vi "SCD - Trigger Sequence Generation - Complete Recipe.vi"(8 "error in":errorcluster, 9 "FPS":dbl=10.0 min=1.0 max=30.0 format="%0.2p", 10 "Modulation Cycles\nAt Each Wavelength":dbl=1.0 min=1.0 max=30.0 step=1.0, 11 "LCVR Voltages":dbl[][](array[numeric])=[[0.5, 0.6, 0.7, 0.8, 0.9]]) -> (0 "error out":errorcluster, 1 "LCVR Relaxtion Time":dbl=200.0 format="%#_13g", 3 "SCD Waveforms (Graph)":waveform(dbl)[](graph)=[{"t0"=timestamp(0 s since 1904-01-01), "dt"=0.000125, "Y"=array[4803 elements]}, {"t0"=timestamp(0 s since 1904-01-01), "dt"=0.000125, "Y"=array[4803 elements]}, {"t0"=timestamp(0 s since 1904-01-01), "dt"=0.000125, "Y"=array[4803 elements]}, {"t0"=timestamp(0 s since 1904-01-01), "dt"=0.000125, "Y"=array[4803 elements]}, {"t0"=timestamp(0 s since 1904-01-01), "dt"=0.000125, "Y"=array[4803 elements]}, {"t0"=timestamp(0 s since 1904-01-01), "dt"=0.000125, "Y"=array[4803 elements]}, {"t0"=timestamp(0 s since 1904-01-01), "dt"=0.000125, "Y"=array[4803 elements]}, {"t0"=timestamp(0 s since 1904-01-01), "dt"=0.000125, "Y"=array[4803 elements]}])   [LabVIEW 2014]
doc: "This VI creates the complete recipe Analog Output waveform set for multiple wavelengths. Each wavelength change in the recipe requies a new 200ms 'relaxation' time for the LCVR's to reach the required retardance value. Finally, this VI pre-pends an Andor Neo Camera \"Arming\" trigger pulse. This is required in a sequence based acquisition."
uses:
  <vilib>/Waveform/WDTOps.llb/WDT Index Channel DBL.vi
  <vilib>/Waveform/WDTOps.llb/WDT Append Waveforms DBL.vi
panel:
  out "SCD Waveforms (cluster)":waveform(dbl)[](array[waveform])=[{"t0"=timestamp(0 s since 1904-01-01), "dt"=0.000125, "Y"=array[4803 elements]}, {"t0"=timestamp(0 s since 1904-01-01), "dt"=0.000125, "Y"=array[4803 elements]}, {"t0"=timestamp(0 s since 1904-01-01), "dt"=0.000125, "Y"=array[4803 elements]}, {"t0"=timestamp(0 s since 1904-01-01), "dt"=0.000125, "Y"=array[4803 elements]}, {"t0"=timestamp(0 s since 1904-01-01), "dt"=0.000125, "Y"=array[4803 elements]}, {"t0"=timestamp(0 s since 1904-01-01), "dt"=0.000125, "Y"=array[4803 elements]}, {"t0"=timestamp(0 s since 1904-01-01), "dt"=0.000125, "Y"=array[4803 elements]}, {"t0"=timestamp(0 s since 1904-01-01), "dt"=0.000125, "Y"=array[4803 elements]}]
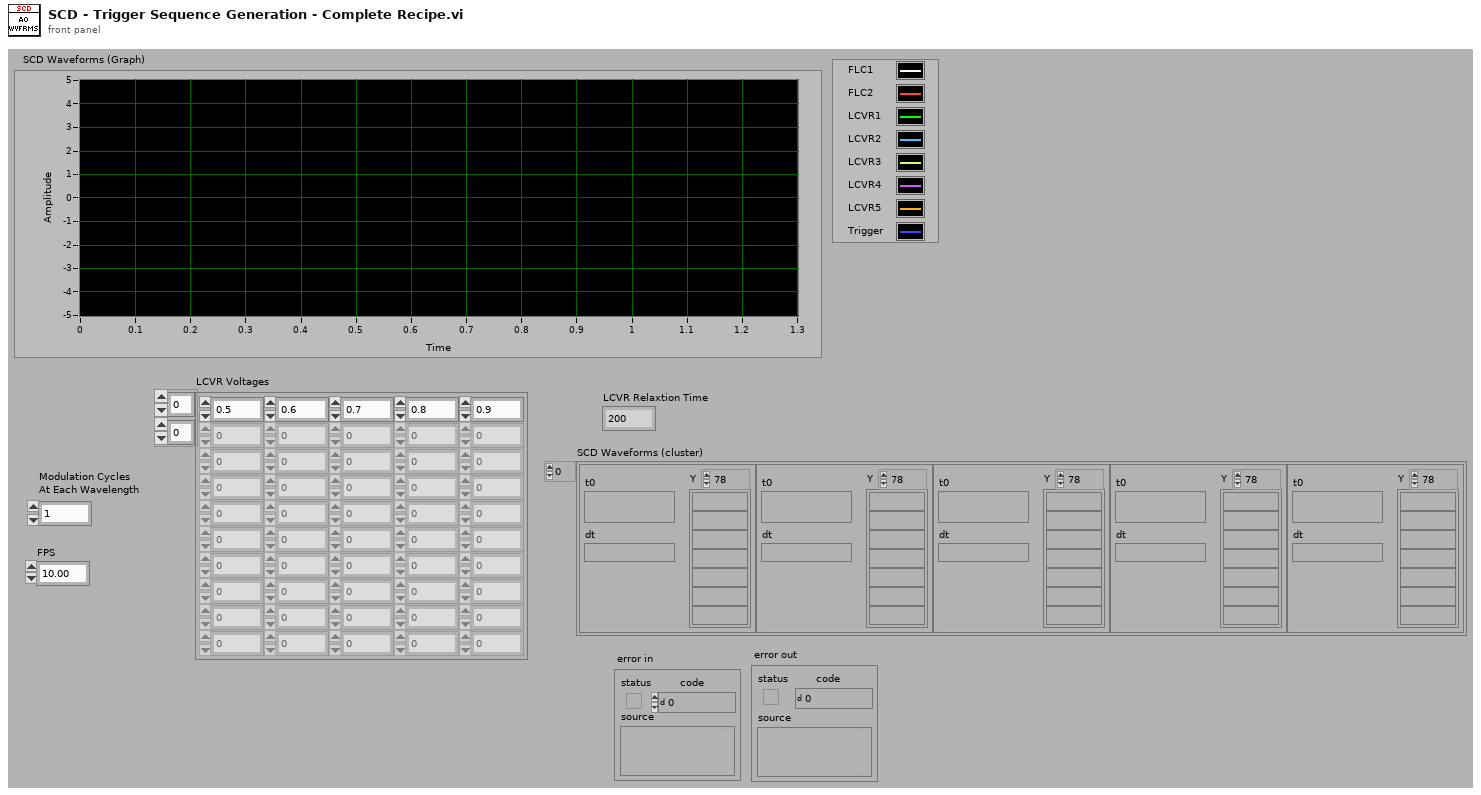
[diagram p1: front panel]
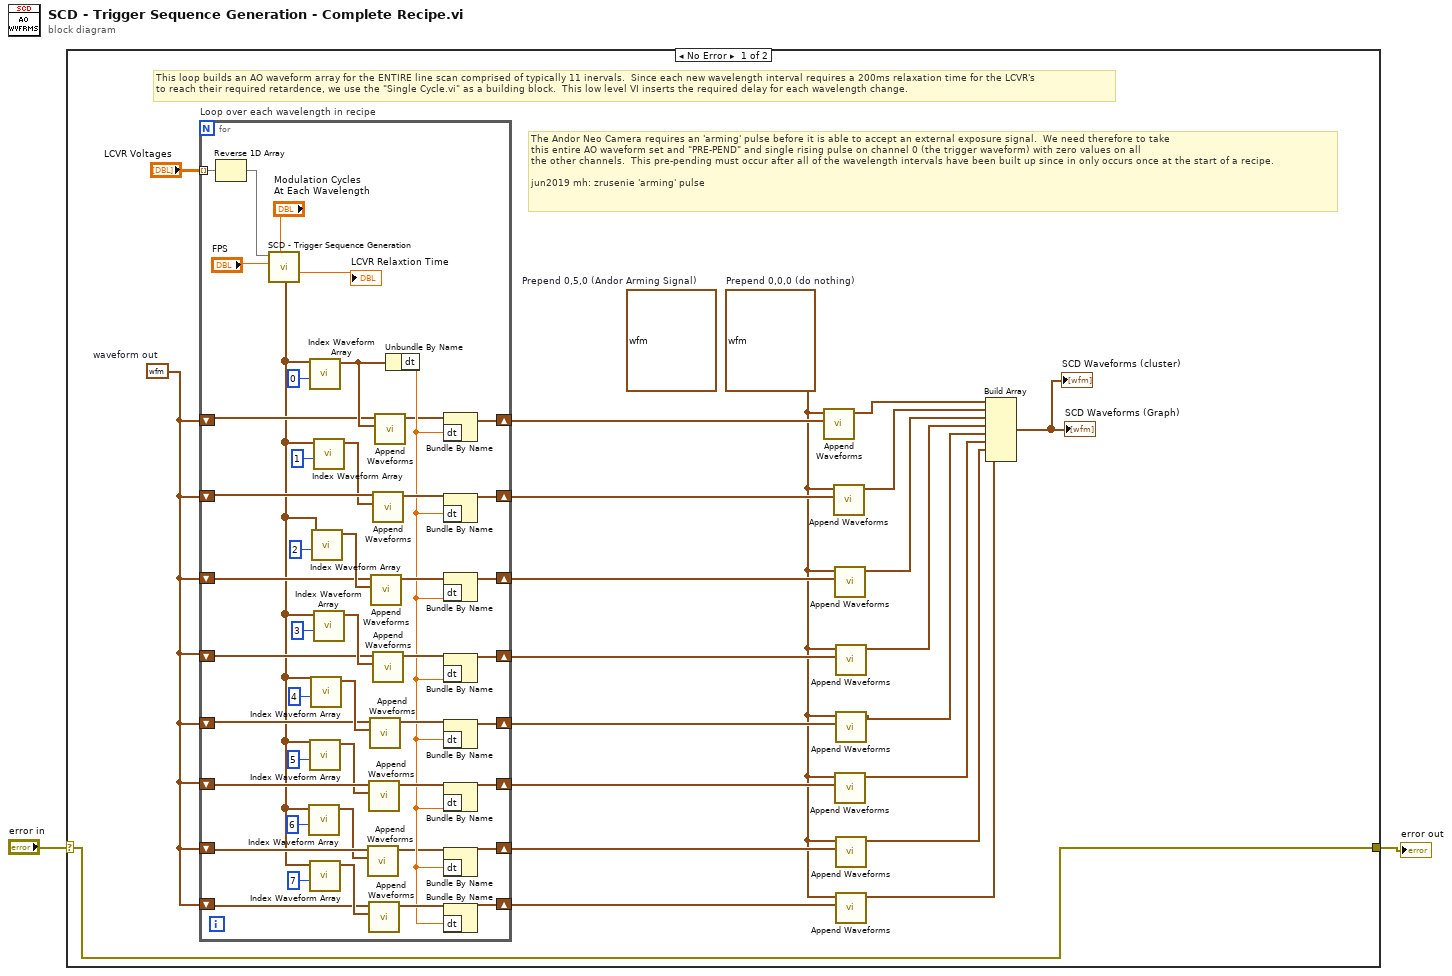
[diagram p0: block diagram]
diagram:
  n1 = case shown="No Error" "error in" {
    selector: "error in" -> [w6 w71]
    tunnel: [w6 w71] -> w1
    frame No Error {
      w3 = waveform(dbl) {"t0"=timestamp(0 s since 1904-01-01), "dt"=0.000125, "Y"=[0.0, 0.0, 0.0]}  # Prepend 0,0,0 (do nothing)
      (unwired) waveform(dbl) {"t0"=timestamp(0 s since 1904-01-01), "dt"=0.000125, "Y"=[0.0, 5.0, 0.0]}  # Prepend 0,5,0 (Andor Arming Signal)
      w23 = waveform(dbl) {"t0"=timestamp(0 s since 1904-01-01), "dt"=1.0, "Y"=[]}  # waveform out
      # "The Andor Neo Camera requires an 'arming' pulse before it is able to accept an external exposure signal.  We need therefore to take\nthis entire AO waveform set and \"PRE-PEND\" and single rising pulse on channel 0 (the trigger waveform) with zero values on all\nthe other channels.  This pre-pending must occur after all of the wavelength intervals have been built up since in only occurs once at the start of a recipe.\n\njun2019 mh: zrusenie 'arming' pulse"
      # "This loop builds an AO waveform array for the ENTIRE line scan comprised of typically 11 inervals.  Since each new wavelength interval requires a 200ms relaxation time for the LCVR's \nto reach their required retardence, we use the \"Single Cycle.vi\" as a building block.  This low level VI inserts the required delay for each wavelength change."
      n2 = for "Loop over each wavelength in recipe" {
        shift-right: [w43] -> w21
        shift-left: w23 -> [w33]
        shift-right: [w27] -> w20
        shift-left: w23 -> [w66]
        shift-right: [w44] -> w18
        shift-left: w23 -> [w53]
        shift-right: [w45] -> w10
        shift-left: w23 -> [w52]
        shift-right: [w46] -> w11
        shift-left: w23 -> [w51]
        shift-right: [w47] -> w15
        shift-left: w23 -> [w50]
        shift-right: [w48] -> w13
        shift-left: w23 -> [w32]
        shift-right: [w38] -> w12
        shift-left: w23 -> [w39]
        tunnel: "LCVR Voltages" -> [w26] mode=indexing
        n3 = Reverse 1D Array(array=w26) -> (reversed array=w36:dbl[])
        n4 = call "SCD - Trigger Sequence Generation.vi"("Modulation Cycles\n per Wavelength"="Modulation Cycles\nAt Each Wavelength", "FPS"="FPS", "LCVR Tuning Voltages"=w36) -> ("LCVR Relaxtion Time (ms)"=→"LCVR Relaxtion Time":dbl, "AO Waveforms"=w24:waveform(dbl)[])  [unwired: 6 in, 1 out]
        n5 = call-poly <vilib>:"Index Waveform Array.vi"("index"=6, "waveform array"=w24) -> ("waveform"=w30:waveform(dbl))  [unwired: 8 in, 1 out]
        n6 = call-poly <vilib>:"Index Waveform Array.vi"("index"=0, "waveform array"=w24) -> ("waveform"=w69:waveform(dbl))  [unwired: 8 in, 1 out]
        n7 = call-poly <vilib>:"Index Waveform Array.vi"("index"=5, "waveform array"=w24) -> ("waveform"=w29:waveform(dbl))  [unwired: 8 in, 1 out]
        n8 = call-poly <vilib>:"Index Waveform Array.vi"("index"=7, "waveform array"=w24) -> ("waveform"=w41:waveform(dbl))  [unwired: 8 in, 1 out]
        n9 = call-poly <vilib>:"Index Waveform Array.vi"("index"=4, "waveform array"=w24) -> ("waveform"=w54:waveform(dbl))  [unwired: 8 in, 1 out]
        n10 = call-poly <vilib>:"Index Waveform Array.vi"("index"=2, "waveform array"=w24) -> ("waveform"=w56:waveform(dbl))  [unwired: 8 in, 1 out]
        n11 = call-poly <vilib>:"Index Waveform Array.vi"("index"=1, "waveform array"=w24) -> ("waveform"=w65:waveform(dbl))  [unwired: 8 in, 1 out]
        n12 = call-poly <vilib>:"Index Waveform Array.vi"("index"=3, "waveform array"=w24) -> ("waveform"=w55:waveform(dbl))  [unwired: 8 in, 1 out]
        n13 = call-poly <vilib>:"Append Waveforms.vi"("waveform B"=w30, "waveform A"=w32) -> ("waveform out"=w31:waveform(dbl))  [unwired: 8 in, 1 out]
        n14 = call-poly <vilib>:"Append Waveforms.vi"("waveform B"=w29, "waveform A"=w50) -> ("waveform out"=w57:waveform(dbl))  [unwired: 8 in, 1 out]
        n15 = call-poly <vilib>:"Append Waveforms.vi"("waveform B"=w41, "waveform A"=w39) -> ("waveform out"=w42:waveform(dbl))  [unwired: 8 in, 1 out]
        n16 = call-poly <vilib>:"Append Waveforms.vi"("waveform B"=w54, "waveform A"=w51) -> ("waveform out"=w59:waveform(dbl))  [unwired: 8 in, 1 out]
        n17 = call-poly <vilib>:"Append Waveforms.vi"("waveform B"=w56, "waveform A"=w53) -> ("waveform out"=w63:waveform(dbl))  [unwired: 8 in, 1 out]
        n18 = call-poly <vilib>:"Append Waveforms.vi"("waveform B"=w65, "waveform A"=w66) -> ("waveform out"=w67:waveform(dbl))  [unwired: 8 in, 1 out]
        n19 = call-poly <vilib>:"Append Waveforms.vi"("waveform B"=w55, "waveform A"=w52) -> ("waveform out"=w61:waveform(dbl))  [unwired: 8 in, 1 out]
        n20 = call-poly <vilib>:"Append Waveforms.vi"("waveform B"=w69, "waveform A"=w33) -> ("waveform out"=w34:waveform(dbl))  [unwired: 8 in, 1 out]
        n21 = Unbundle By Name(w69) -> ("dt"=w40:dbl)
        n22 = Bundle By Name(cluster=w34, "dt"=w40) -> (w43:waveform(dbl))
        n23 = Bundle By Name(cluster=w67, "dt"=w40) -> (w27:waveform(dbl))
        n24 = Bundle By Name(cluster=w63, "dt"=w40) -> (w44:waveform(dbl))
        n25 = Bundle By Name(cluster=w61, "dt"=w40) -> (w45:waveform(dbl))
        n26 = Bundle By Name(cluster=w59, "dt"=w40) -> (w46:waveform(dbl))
        n27 = Bundle By Name(cluster=w57, "dt"=w40) -> (w47:waveform(dbl))
        n28 = Bundle By Name(cluster=w31, "dt"=w40) -> (w48:waveform(dbl))
        n29 = Bundle By Name(cluster=w42, "dt"=w40) -> (w38:waveform(dbl))
      }
      n30 = call-poly <vilib>:"Append Waveforms.vi"("waveform B"=w21, "waveform A"=w3) -> ("waveform out"=w4:waveform(dbl))  [unwired: 8 in, 1 out]
      n31 = call-poly <vilib>:"Append Waveforms.vi"("waveform B"=w20, "waveform A"=w3) -> ("waveform out"=w19:waveform(dbl))  [unwired: 8 in, 1 out]
      n32 = call-poly <vilib>:"Append Waveforms.vi"("waveform B"=w18, "waveform A"=w3) -> ("waveform out"=w17:waveform(dbl))  [unwired: 8 in, 1 out]
      n33 = call-poly <vilib>:"Append Waveforms.vi"("waveform B"=w15, "waveform A"=w3) -> ("waveform out"=w14:waveform(dbl))  [unwired: 8 in, 1 out]
      n34 = call-poly <vilib>:"Append Waveforms.vi"("waveform B"=w10, "waveform A"=w3) -> ("waveform out"=w16:waveform(dbl))  [unwired: 8 in, 1 out]
      n35 = call-poly <vilib>:"Append Waveforms.vi"("waveform B"=w11, "waveform A"=w3) -> ("waveform out"=w9:waveform(dbl))  [unwired: 8 in, 1 out]
      n36 = call-poly <vilib>:"Append Waveforms.vi"("waveform B"=w13, "waveform A"=w3) -> ("waveform out"=w8:waveform(dbl))  [unwired: 8 in, 1 out]
      n37 = call-poly <vilib>:"Append Waveforms.vi"("waveform B"=w12, "waveform A"=w3) -> ("waveform out"=w7:waveform(dbl))  [unwired: 8 in, 1 out]
      n38 = Build Array(w4, w19, w17, w16, w9, w14, w8, w7) -> (→"SCD Waveforms (Graph)" →"SCD Waveforms (cluster)":waveform(dbl)[])
    }
    frame Error {
    }
  }
  "error out" <- w1
